vi "New Image Threshold.vi"(8 "error in (no error)":errorcluster, 10 "New Image":T1, 11 "Threshold in":refnum<class "Threshold.lvclass">) -> (0 "error out":errorcluster, 3 "Threshold out":refnum<class "Threshold.lvclass">)   [LabVIEW 2016, in "Tests.lvlib" / "Threshold.lvclass"]
uses:
  Threshold.lvclass
  <vilib>/vision/Image Controls.llb/IMAQ Image.ctl
  Threshold.lvclass/Threshold.ctl
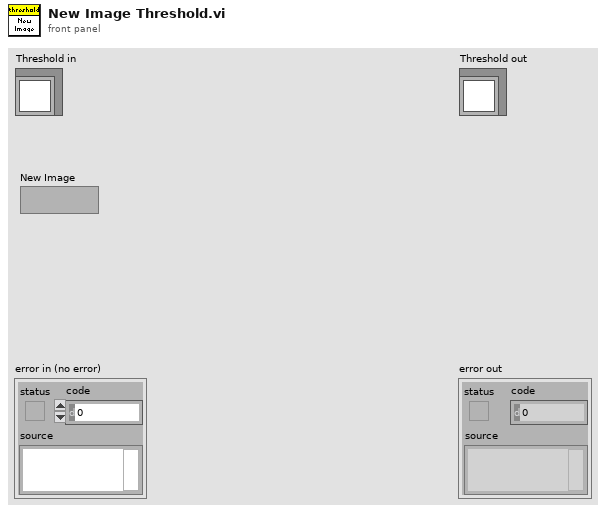
[diagram p1: front panel]
types:
  T1 = typedef "IMAQ Image.ctl" = refnum<image>
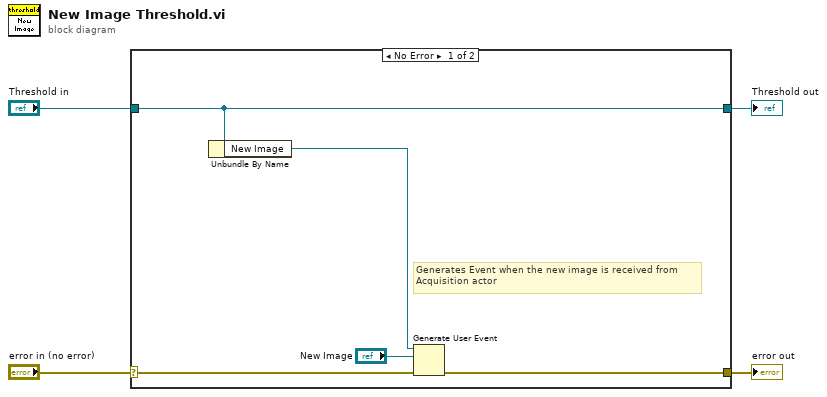
[diagram p0: block diagram]
diagram:
  n1 = case shown="No Error" "error in (no error)" {
    selector: "error in (no error)" -> [w8 w11]
    tunnel: [w7 w11] -> w3
    tunnel: [w9 w10] -> w1
    tunnel: "Threshold in" -> [w9 w10]
    frame No Error {
      # "Generates Event when the new image is received from\nAcquisition actor"
      n2 = Unbundle By Name(w9) -> ("New Image"=w6:refnum<user-event>)
      n3 = Generate User Event(user event=w6, event data cluster="New Image", error in=w8) -> (error out=w7:errorcluster)  [unwired: 1 in, 1 out]
    }
    frame Error {
    }
  }
  "error out" <- w3
  "Threshold out" <- w1
